vi "Compare Log Records.vi"(6 "ignore data? (F)":bool, 8 "expected data":variant, 9 "expected message":string, 10 "expected log level":T2, 11 "log record":T1 {"timestamp" format="%<%x %.3X>T"}) -> (3 "match?":bool)   [LabVIEW 2018]
uses:
  Logger/Internal Log Levels.ctl
  Log Record.ctl
  Logging.lvlib
panel:
  # "Connector Pane"
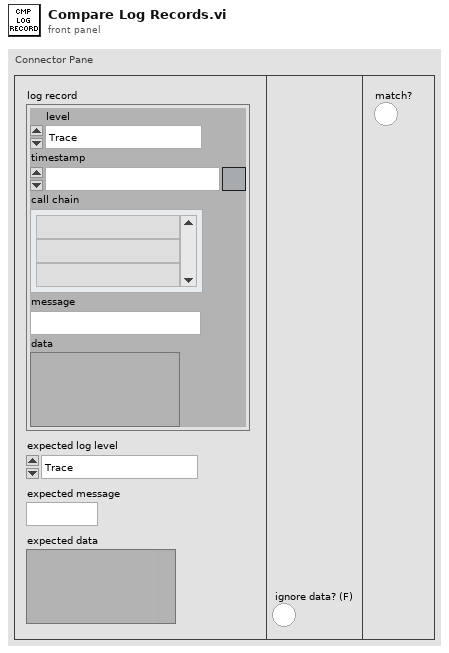
[diagram p1: front panel]
types:
  T1 = typedef "Logging.lvlib/Log Record.ctl" = cluster{"level":T2, "timestamp":timestamp, "call chain":string[], "message":string, "data":variant}
  T2 = typedef "Logging.lvlib/Internal Log Levels.ctl" = enum16{"Trace", "Debug", "Info", "Warning", "Error", "Critical", "Internal"}
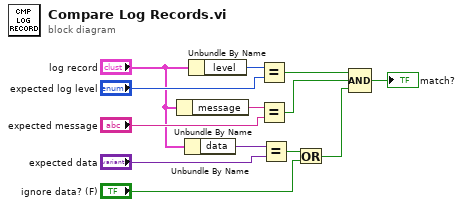
[diagram p0: block diagram]
diagram:
  n1 = Unbundle By Name("log record") -> ("message"=w11:string)
  n2 = Unbundle By Name("log record") -> ("data"=w8:variant)
  n3 = Unbundle By Name("log record") -> ("level"=w13:T2)
  n4 = Equal?(x=w13, y="expected log level") -> (x = y?=w6:bool)
  n5 = Equal?(x=w11, y="expected message") -> (x = y?=w5:bool)
  n6 = Equal?(x=w8, y="expected data") -> (x = y?=w4:bool)
  n7 = Or(x=w4, y="ignore data? (F)") -> (x .or. y?=w2:bool)
  n8 = Compound Arithmetic op=AND(w6, w5, w2) -> (→"match?":bool)
